vi "Set Stream State.vi"(8 "error in (no error)":errorcluster, 9 "stream state":T1, 10 "stream index":i32, 11 "refnum in":refnum<k20>) -> (0 "error out":errorcluster, 3 "refnum out":refnum<k20>)   [LabVIEW 2015, in "niInstr Streaming v1 Host.lvlib"]
doc: "Sets the requested stream state using the FPGA host interface.\n\n<B>Input Parameters</B>\n\n<B>error in (no error)</B> 'error in' can accept error information wired from VIs previously called. Use this information to decide if any functionality should be bypassed in the event of errors from other VIs.\n\nRight-click the 'error in' control on the front panel and select 'Explain Error' or 'Explain Warning' from the shortcut menu for more information about the error.\n\n<B>stream index</B> Selects which stream index this VI will interface to. This is the index number at the end of the host interface controls (0..7).\n\n<B>refnum in</B> Wire in the session obtained from Open FPGA Reference.\n\n<B>Output Parameters</B>\n\n<B>error out</B> contains error information. This output provides standard error out functionality.\n\n<B>refnum out</B> Copy of refnum in"
uses:
  <instrlib>/_niInstr/Streaming/v1/Host/niInstr Streaming v1 Host.lvlib
  <instrlib>/_niInstr/Streaming/v1/Common/Stream State.ctl
  <instrlib>/_niInstr/Streaming/v1/Host/Public/Stream Host Interface.ctl
  <vilib>/Utility/error.llb/Error Cluster From Error Code.vi
  <vilib>/rvi/errors/niLvFpgaAdjustHostInterfaceError.vi
  <vilib>/ErrorRing/Error Ring.xnode
  <vilib>/rvi/interface/nirviReadWriteControl/nirviReadWriteControl.xnode
  NiFpgaLv.dll
  <vilib>/rvi/interface/Simulation/niFpgaSimulationCallBeginRW.vi
  <instrlib>/_niInstr/Streaming/v1/Common/niInstr Streaming v1 Common.lvlib
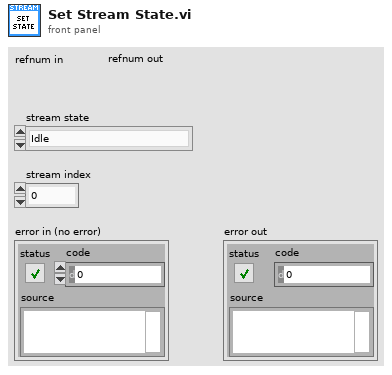
[diagram p1: front panel]
types:
  T1 = typedef "niInstr Streaming v1 Common.lvlib/Stream State.ctl" = enum8{"Idle", "Finite Transfer", "Continuous", "Done", "Error", "Not Ready", "Cancel"}
  T2 = typedef "niInstr Streaming v1 Host.lvlib/Stream Host Interface.ctl" = refnum<k20>
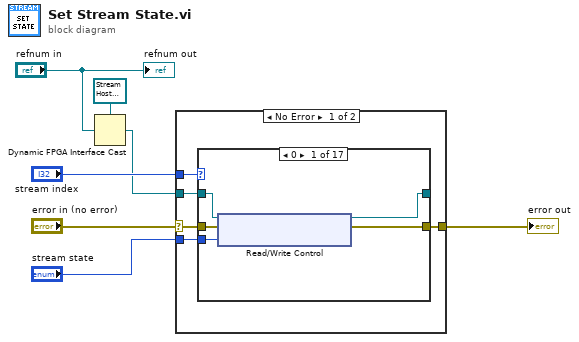
[diagram p0: block diagram]
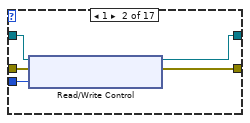
[diagram p2: hidden frame]
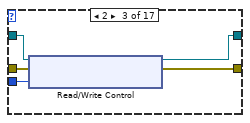
[diagram p3: hidden frame]
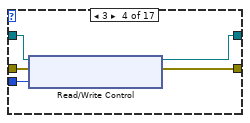
[diagram p4: hidden frame]
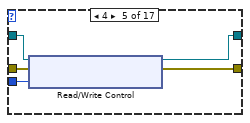
[diagram p5: hidden frame]
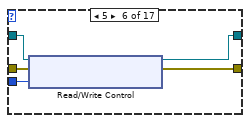
[diagram p6: hidden frame]
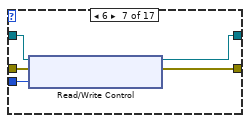
[diagram p7: hidden frame]
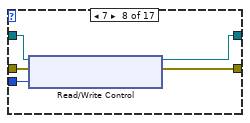
[diagram p8: hidden frame]
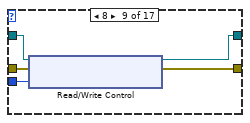
[diagram p9: hidden frame]
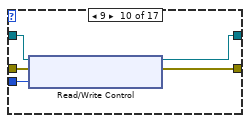
[diagram p10: hidden frame]
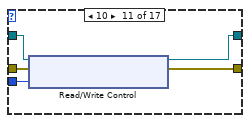
[diagram p11: hidden frame]
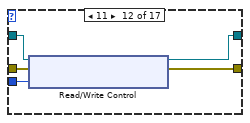
[diagram p12: hidden frame]
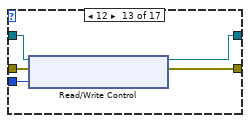
[diagram p13: hidden frame]
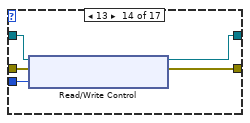
[diagram p14: hidden frame]
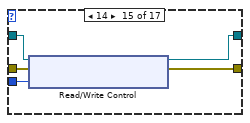
[diagram p15: hidden frame]
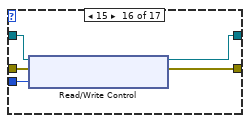
[diagram p16: hidden frame]
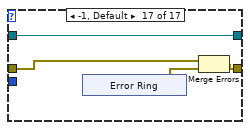
[diagram p17: hidden frame]
diagram:
  n1 = Dynamic FPGA Interface Cast(Session In=T2 refnum ("Refnum in"), Type="refnum in") -> (Session Out=w2:T2)
  n2 = case shown="No Error" "error in (no error)" {
    selector: "error in (no error)" -> [w8 w101]
    tunnel: "stream index" -> [w12 _]
    tunnel: "stream state" -> [w11 _]
    tunnel: [w10 w101] -> w5
    tunnel: w2 -> [w9 _]
    frame No Error {
      n3 = case shown="0" w12 {
        tunnel: w8 -> [w17 w22 w27 w32 w37 w42 w47 w52 w57 w62 w67 w72 w77 w82 w87 w92 w94]
        tunnel: w11 -> [w16 w21 w26 w31 w36 w41 w46 w51 w56 w61 w66 w71 w76 w81 w86 w91 _]
        tunnel: [w15 w20 w25 w30 w35 w40 w45 w50 w55 w60 w65 w70 w75 w80 w85 w90 w96] -> _
        tunnel: [w14 w19 w24 w29 w34 w39 w44 w49 w54 w59 w64 w69 w74 w79 w84 w89 w95] -> w10
        tunnel: w9 -> [w13 w18 w23 w28 w33 w38 w43 w48 w53 w58 w63 w68 w73 w78 w83 w88 w96]
        frame 0 {
          n4 = xnode "Read/Write Control"("FPGA VI Reference In"=w13, "error in"=w17, "stream.request state 0"=w16) -> ("FPGA VI Reference Out"=w15:T2, "error out"=w14:errorcluster)
        }
        frame 1 {
          n5 = xnode "Read/Write Control"("FPGA VI Reference In"=w18, "error in"=w22, "stream.request state 1"=w21) -> ("FPGA VI Reference Out"=w20:T2, "error out"=w19:errorcluster)
        }
        frame 2 {
          n6 = xnode "Read/Write Control"("FPGA VI Reference In"=w23, "error in"=w27, "stream.request state 2"=w26) -> ("FPGA VI Reference Out"=w25:T2, "error out"=w24:errorcluster)
        }
        frame 3 {
          n7 = xnode "Read/Write Control"("FPGA VI Reference In"=w28, "error in"=w32, "stream.request state 3"=w31) -> ("FPGA VI Reference Out"=w30:T2, "error out"=w29:errorcluster)
        }
        frame 4 {
          n8 = xnode "Read/Write Control"("FPGA VI Reference In"=w33, "error in"=w37, "stream.request state 4"=w36) -> ("FPGA VI Reference Out"=w35:T2, "error out"=w34:errorcluster)
        }
        frame 5 {
          n9 = xnode "Read/Write Control"("FPGA VI Reference In"=w38, "error in"=w42, "stream.request state 5"=w41) -> ("FPGA VI Reference Out"=w40:T2, "error out"=w39:errorcluster)
        }
        frame 6 {
          n10 = xnode "Read/Write Control"("FPGA VI Reference In"=w43, "error in"=w47, "stream.request state 6"=w46) -> ("FPGA VI Reference Out"=w45:T2, "error out"=w44:errorcluster)
        }
        frame 7 {
          n11 = xnode "Read/Write Control"("FPGA VI Reference In"=w48, "error in"=w52, "stream.request state 7"=w51) -> ("FPGA VI Reference Out"=w50:T2, "error out"=w49:errorcluster)
        }
        frame 8 {
          n12 = xnode "Read/Write Control"("FPGA VI Reference In"=w53, "error in"=w57, "stream.request state 8"=w56) -> ("FPGA VI Reference Out"=w55:T2, "error out"=w54:errorcluster)
        }
        frame 9 {
          n13 = xnode "Read/Write Control"("FPGA VI Reference In"=w58, "error in"=w62, "stream.request state 9"=w61) -> ("FPGA VI Reference Out"=w60:T2, "error out"=w59:errorcluster)
        }
        frame 10 {
          n14 = xnode "Read/Write Control"("FPGA VI Reference In"=w63, "error in"=w67, "stream.request state 10"=w66) -> ("FPGA VI Reference Out"=w65:T2, "error out"=w64:errorcluster)
        }
        frame 11 {
          n15 = xnode "Read/Write Control"("FPGA VI Reference In"=w68, "error in"=w72, "stream.request state 11"=w71) -> ("FPGA VI Reference Out"=w70:T2, "error out"=w69:errorcluster)
        }
        frame 12 {
          n16 = xnode "Read/Write Control"("FPGA VI Reference In"=w73, "error in"=w77, "stream.request state 12"=w76) -> ("FPGA VI Reference Out"=w75:T2, "error out"=w74:errorcluster)
        }
        frame 13 {
          n17 = xnode "Read/Write Control"("FPGA VI Reference In"=w78, "error in"=w82, "stream.request state 13"=w81) -> ("FPGA VI Reference Out"=w80:T2, "error out"=w79:errorcluster)
        }
        frame 14 {
          n18 = xnode "Read/Write Control"("FPGA VI Reference In"=w83, "error in"=w87, "stream.request state 14"=w86) -> ("FPGA VI Reference Out"=w85:T2, "error out"=w84:errorcluster)
        }
        frame 15 {
          n19 = xnode "Read/Write Control"("FPGA VI Reference In"=w88, "error in"=w92, "stream.request state 15"=w91) -> ("FPGA VI Reference Out"=w90:T2, "error out"=w89:errorcluster)
        }
        frame -1, Default {
          n20 = xnode "Error Ring"() -> ("error out"=w93:errorcluster)
          n21 = Merge Errors(w94, w93) -> (w95:errorcluster)
        }
      }
    }
    frame Error {
    }
  }
  "error out" <- w5
  "refnum out" <- "refnum in"
